vi "Attitude_Display.vi"() -> ()   [LabVIEW 2013]
uses:
  <vilib>/robotics/Controls/Attitude Indicator/Attitude Indicator.xctl
  <vilib>/Utility/file.llb/Read From Spreadsheet File (DBL).vi
panel:
  out "x-y":u32
  in  "Stop Button":bool
  out "output cluster":cluster{"first row[0]":dbl, "first row[1]":dbl}
  out "Attitude Indicator":cluster{"Roll":dbl, "Pitch":dbl}(xcontrol)
  in  "Spreadsheet path (.csv) 2":path=path "C:/Users/husmith/Desktop/MyData.csv"
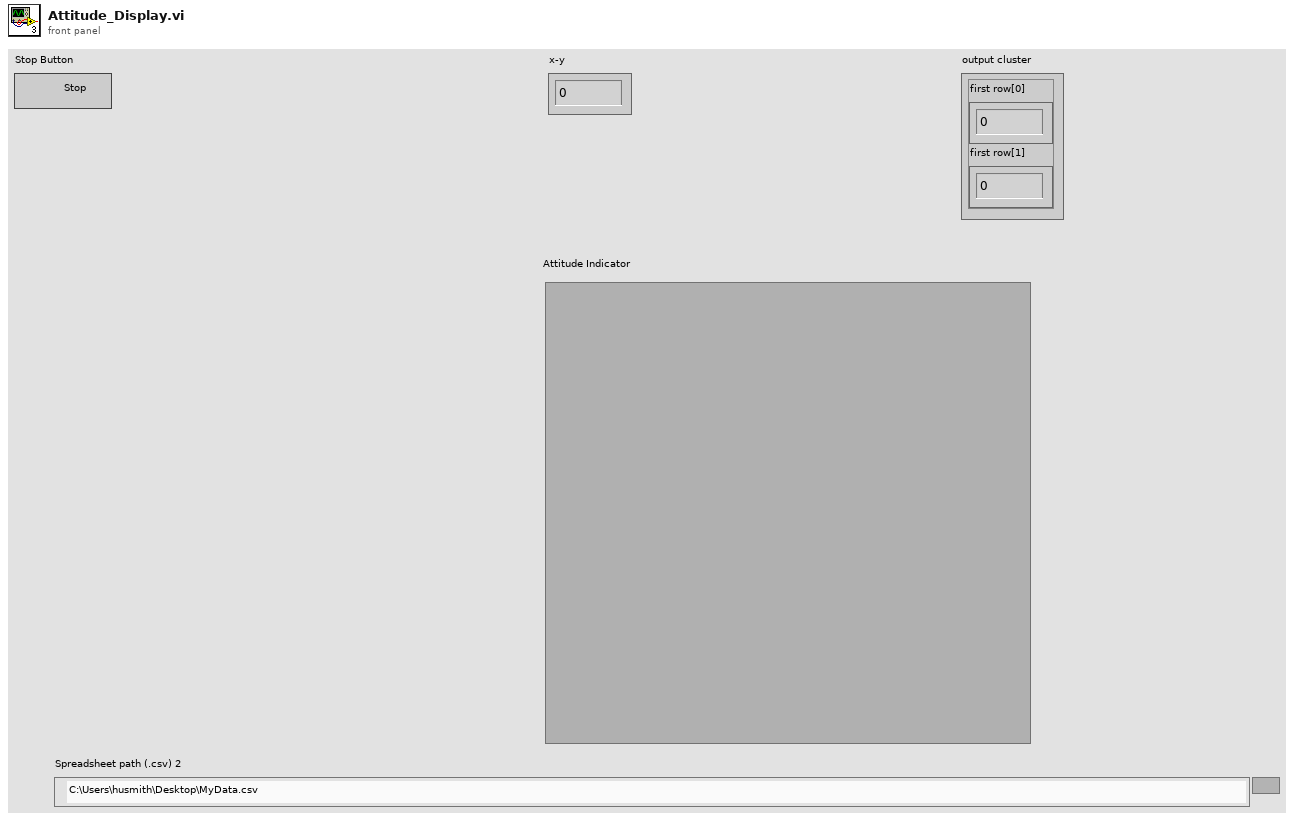
[diagram p1: front panel]
types:
  T1 = cluster{"all rows[0]":dbl, "all rows[1]":dbl, "all rows[2]":dbl, "all rows[3]":dbl, "all rows[4]":dbl, "all rows[5]":dbl, "all rows[6]":dbl, "all rows[7]":dbl, "all rows[8]":dbl}
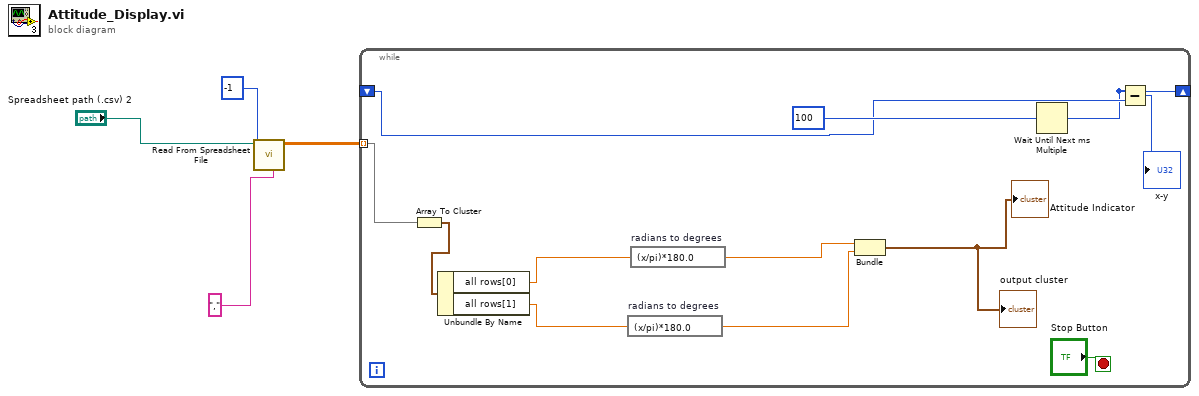
[diagram p0: block diagram]
diagram:
  n1 = call-poly <vilib>:"Read From Spreadsheet File.vi"("delimiter (\\t)"="," ("delimiter (\\t)"), "number of rows (all:-1)"=-1, "file path (dialog if empty)"="Spreadsheet path (.csv) 2") -> ("all rows"=w2:dbl[][])  [unwired: 4 in, 4 out]
  n2 = while {
    tunnel: w2 -> [w14] mode=indexing
    shift-right: [w6] -> _
    shift-left: _ -> [w7]
    stop <- "Stop Button" stop-if-true
    n3 = Array To Cluster(array=w14) -> (cluster=w15:T1)
    n4 = Unbundle By Name(w15) -> ("all rows[0]"=w11:dbl, "all rows[1]"=w9:dbl)
    n5 = expression code="(x/pi)*180.0" "radians to degrees"(w9) -> (w8:dbl)
    n6 = expression code="(x/pi)*180.0" "radians to degrees"(w11) -> (w10:dbl)
    n7 = Bundle("all rows[0]"=w10, "all rows[1]"=w8) -> (→"Attitude Indicator" →"output cluster":cluster{"all rows[0]":dbl, "all rows[1]":dbl})  [unwired: 1 in]
    n8 = Wait Until Next ms Multiple(millisecond multiple=u32 100) -> (millisecond timer value=w6:u32)
    n9 = Subtract(x=w6, y=w7) -> (x-y=→"x-y":u32)
  }
